vi "Read Caller VI Refnum.vi"(8 "error in (no error)":errorcluster, 11 "UI ActorTop in":refnum<class "UIActorTop.lvclass">) -> (0 "error out":errorcluster, 2 "Caller VI Refnum":refnum<vi>, 3 "UI ActorTop out":refnum<class "UIActorTop.lvclass">)   [LabVIEW 2021, in "AbstractActorTemplate.lvlib" / "UIActorTop.lvclass"]
uses:
  <userlib>/John_Lib/AbstractActorTemplate/AbstractActorTemplate/UIActorTop.lvclass
  <userlib>/John_Lib/AbstractActorTemplate/AbstractActorTemplate/UIActorTop.lvclass/UIActorTop.ctl
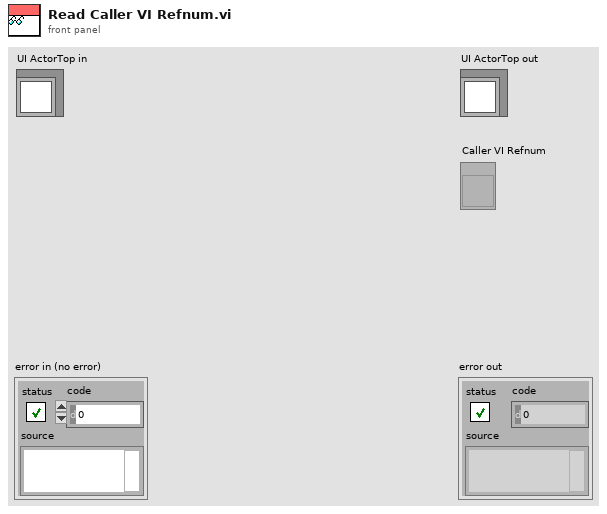
[diagram p1: front panel]
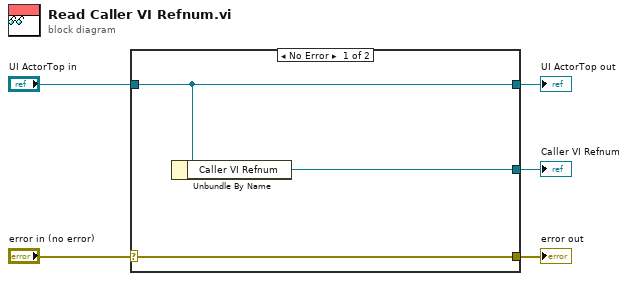
[diagram p0: block diagram]
diagram:
  n1 = case shown="No Error" "error in (no error)" {
    selector: "error in (no error)" -> [w8 w9]
    tunnel: [w8 w9] -> w4
    tunnel: [w7 w10] -> w2
    tunnel: "UI ActorTop in" -> [w7 w10]
    tunnel: [w6 _] -> w1
    frame No Error {
      n2 = Unbundle By Name(w7) -> ("Caller VI Refnum"=w6:refnum<vi>)
    }
    frame Error {
    }
  }
  "error out" <- w4
  "UI ActorTop out" <- w2
  "Caller VI Refnum" <- w1
